vi "TDK3034.vi"() -> ()   [LabVIEW 2013]
panel:
  out "Run info":string caption="String"
  in  "Save Button":bool
  in  "Get Waveform Button":bool
  in  "Serial Configuration":T1={"Baud Rate"=9600, "Parity"=0, "Data Bits"=8, "Stop Bits"=10, "Flow Control"=2} {"Flow Control" items=["None", "XON/XOFF", "RTS/CTS", "XON/XOFF & RTS/CTS", "DTR/DSR", "XON/XOFF & DTR/DSR"]; "Stop Bits" items=["1.0"=10, "1.5"=15, "2.0"=20]; "Data Bits" items=["7"=7, "8"=8]; "Parity" items=["None", "Odd", "Even", "Mark", "Space"]; "Baud Rate" items=["300"=300, "600"=600, "1200"=1200, "2400"=2400, "4800"=4800, "9600"=9600, "19200"=19200]}
  out "Waveform Data":waveform(dbl)(graph)
  in  "Maximum Time (10000 ms)":u32=10000
  in  "Channel (1: Channel 1)":string(combo)
  in  "VISA resource name":refnum<visa-resource-name>
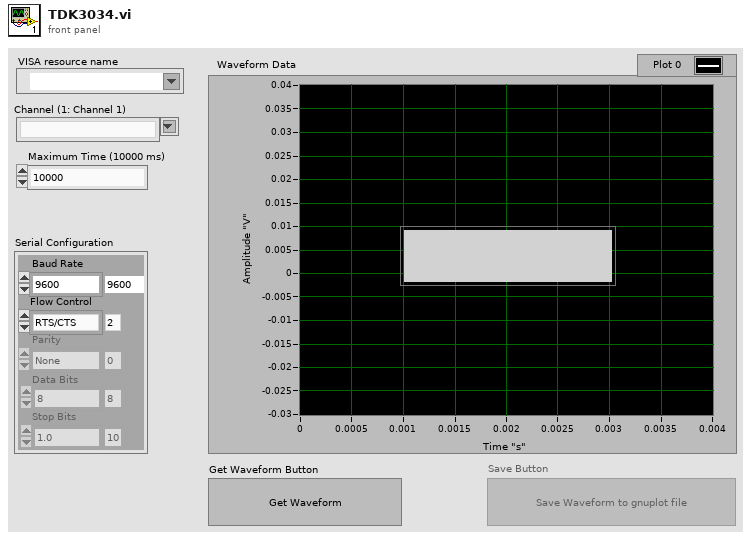
[diagram p1: front panel]
types:
  T1 = cluster{"Baud Rate":u32, "Parity":u16, "Data Bits":u16, "Stop Bits":u16, "Flow Control":u16}
  T2 = enum8{"Enabled", "Disabled", "Disabled and Grayed Out"}
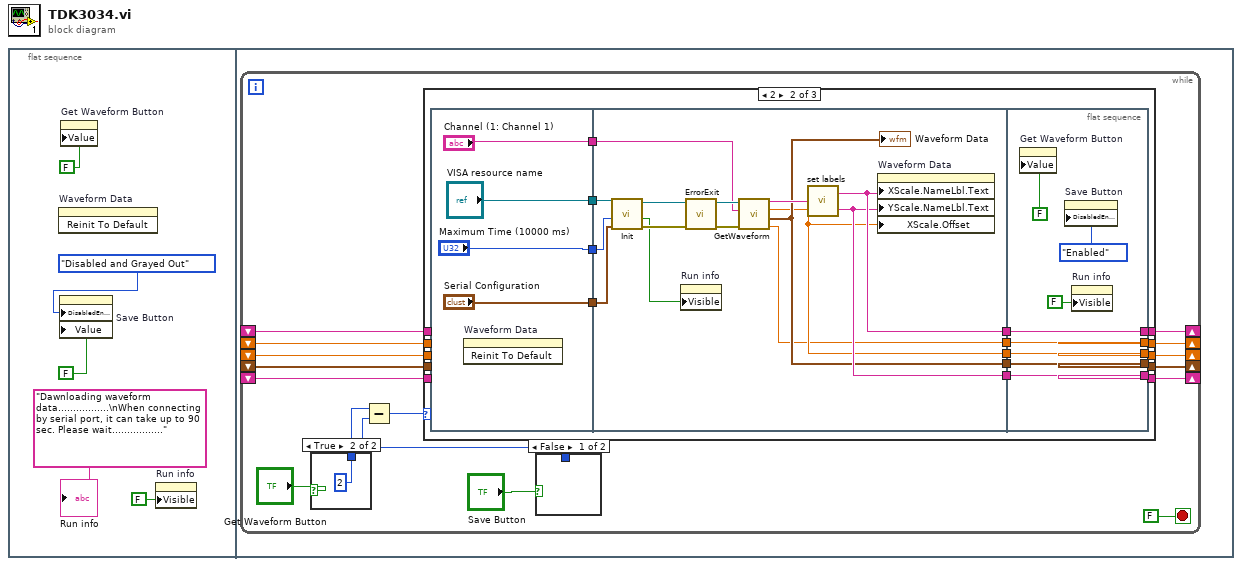
[diagram p0: block diagram]
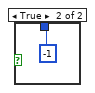
[diagram p2: hidden frame]
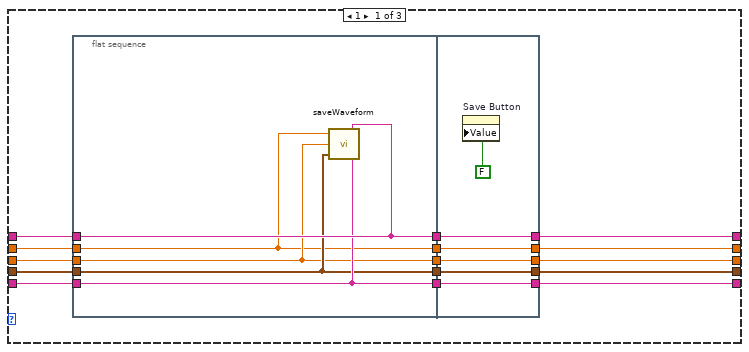
[diagram p4: hidden frame]
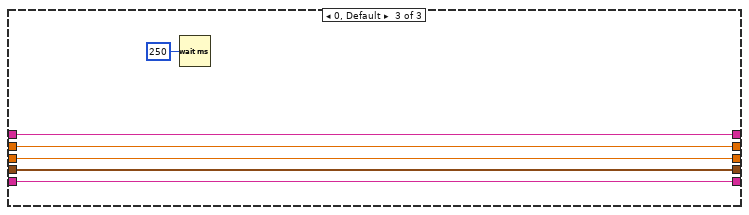
[diagram p5: hidden frame]
diagram:
  n1 = flat-sequence {
    frame #0 {
      n2 = invoke on="Waveform Data" class="WFGraph (strict)" method="Reinit To Default"() -> ()  [unwired: 3 in, 3 out]
      n3 = property on="Save Button" class="Bool (strict)"("DisabledEnum"=T2."Disabled and Grayed Out" ("Disabled"), "Value"=FALSE) -> ()  [unwired: 2 in, 2 out]
      n4 = property on="Get Waveform Button" class="Bool (strict)"("Value"=FALSE ("Get Waveform Button")) -> ()  [unwired: 2 in, 2 out]
      n5 = property on="Run info" class="Str"("Visible"=FALSE) -> ()  [unwired: 2 in, 2 out]
      "Run info" <- "Dawnloading waveform data.................\nWhen connecting by serial port, it can take up to 90 sec. Please wait................." ("Run info")
    }
    frame #1 {
      n6 = while {
        shift-right: [w15] -> _
        shift-left: _ -> [w10]
        shift-right: [w13] -> _
        shift-left: _ -> [w7]
        shift-right: [w11] -> _
        shift-left: _ -> [w9]
        shift-right: [w12] -> _
        shift-left: _ -> [w8]
        shift-right: [w14] -> _
        shift-left: _ -> [w6]
        stop <- FALSE stop-if-true
        n7 = case shown="True" "Get Waveform Button" {
          tunnel: [_ 2] -> w16
          frame False {
          }
          frame True {
          }
        }
        n8 = case shown="False" "Save Button" {
          tunnel: [_ -1] -> w20
          frame False {
          }
          frame True {
          }
        }
        n9 = Subtract(x=w16, y=w20) -> (x-y=w21:i32)
        n10 = case shown="2" w21 {
          tunnel: [w38 w63 w95] -> w15
          tunnel: [w26 w61 w91] -> w14
          tunnel: [w29 w59 w92] -> w13
          tunnel: [w32 w57 w93] -> w12
          tunnel: [w35 w55 w94] -> w11
          tunnel: w10 -> [w36 _ w95]
          tunnel: w9 -> [w33 _ w94]
          tunnel: w8 -> [w30 _ w93]
          tunnel: w7 -> [w27 _ w92]
          tunnel: w6 -> [w24 _ w91]
          frame 1 {
            n11 = flat-sequence {
              tunnel: [w43] -> w37
              tunnel: w36 -> [w43]
              tunnel: [w39] -> w34
              tunnel: w33 -> [w39]
              tunnel: [w40] -> w31
              tunnel: w30 -> [w40]
              tunnel: [w41] -> w28
              tunnel: w27 -> [w41]
              tunnel: [w42] -> w25
              tunnel: w24 -> [w42]
              tunnel: [w48] -> w38
              tunnel: w37 -> [w48]
              tunnel: [w47] -> w35
              tunnel: w34 -> [w47]
              tunnel: [w46] -> w32
              tunnel: w31 -> [w46]
              tunnel: [w45] -> w29
              tunnel: w28 -> [w45]
              tunnel: [w44] -> w26
              tunnel: w25 -> [w44]
              frame #0 {
                n12 = call "saveWaveform.vi"("axe y label"=w42, "axe x label"=w43, "Waveform"=w41, "x_zero"=w40, "pt_off"=w39) -> ()
              }
              frame #1 {
                n13 = property on="Save Button" class="Bool (strict)"("Value"=FALSE ("Save Button")) -> ()  [unwired: 2 in, 2 out]
              }
            }
          }
          frame 2 {
            n14 = flat-sequence {
              tunnel: ["VISA resource name"] -> w53
              tunnel: ["Serial Configuration"] -> w52
              tunnel: ["Channel (1: Channel 1)"] -> w51
              tunnel: ["Maximum Time (10000 ms)"] -> w50
              tunnel: [w73] -> w62
              tunnel: [w72] -> w60
              tunnel: [w71] -> w58
              tunnel: [w70] -> w56
              tunnel: [w69] -> w54
              tunnel: w53 -> [w76]
              tunnel: w52 -> [w74]
              tunnel: w51 -> [w77]
              tunnel: w50 -> [w75]
              tunnel: [w88] -> w63
              tunnel: w62 -> [w88]
              tunnel: [w87] -> w61
              tunnel: w60 -> [w87]
              tunnel: [w86] -> w59
              tunnel: w58 -> [w86]
              tunnel: [w85] -> w57
              tunnel: w56 -> [w85]
              tunnel: [w84] -> w55
              tunnel: w54 -> [w84]
              frame #0 {
                n15 = invoke on="Waveform Data" class="WFGraph (strict)" method="Reinit To Default"() -> ()  [unwired: 3 in, 3 out]
              }
              frame #1 {
                n16 = call "Init.vi"("Serial Configuration"=w74, "General Settings:Timeout Value"=w75, "VISA Refnum in"=w76) -> ("error out"=w78:errorcluster, "serial?"=w68:bool, "VISA Refnum out"=w79:refnum<visa-resource-name>)  [unwired: 6 in]
                n17 = property on="Run info" class="Str"("Visible"=w68) -> ()  [unwired: 2 in, 2 out]
                n18 = call "ErrorExit.vi"("error in (no error)"=w78, "VISA Refnum in"=w79) -> ("error out"=w81:errorcluster, "VISA Refnum out"=w80:refnum<visa-resource-name>)  [unwired: 8 in]
                n19 = call "GetWaveform.vi"("error in (no error)"=w81, "Channel (1: Channel 1)"=w77, "VISA Refnum in"=w80) -> ("pt_off"=w69:dbl, "Waveform"=w71:waveform(dbl), "x_zero"=w70:dbl, "axis labels"=w82:string)  [unwired: 5 in]
                "Waveform Data" <- w71
                n20 = call "set labels.vi"("axis labels"=w82) -> ("axe x label"=w73:string, "axe y label"=w72:string)
                n21 = property on="Waveform Data" class="WFGraph (strict)"("XScale.NameLbl.Text"=w73, "YScale.NameLbl.Text"=w72, "XScale.Offset"=w70) -> ()  [unwired: 2 in, 2 out]
              }
              frame #2 {
                n22 = property on="Get Waveform Button" class="Bool (strict)"("Value"=FALSE ("Get Waveform Button")) -> ()  [unwired: 2 in, 2 out]
                n23 = property on="Save Button" class="Bool (strict)"("DisabledEnum"=T2."Enabled" ("Disabled")) -> ()  [unwired: 2 in, 2 out]
                n24 = property on="Run info" class="Str"("Visible"=FALSE) -> ()  [unwired: 2 in, 2 out]
              }
            }
          }
          frame 0, Default {
            n25 = Wait (ms)(milliseconds to wait=u32 250) -> ()  [unwired: 1 out]
          }
        }
      }
    }
  }
